vi "tdmstest.vi"   [LabVIEW 2019]
uses:
  TDMSLogger_class/TDMSLogger.lvclass
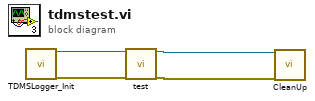
[diagram p0: block diagram]
diagram:
  n1 = call "TDMSLogger_Init.vi"() -> ("object out"=w4:refnum<class "TDMSLogger.lvclass">, "error out"=w3:errorcluster)  [unwired: 17 in, 1 out]
  n2 = call-dynamic "test.vi"("object in"=w4, "error in (no error)"=w3) -> ("object out"=w2:refnum<class "TDMSLogger.lvclass">, "error out"=w1:errorcluster)  [unwired: 16 in]
  n3 = call-dynamic "CleanUp.vi"("object in"=w2, "error in (no error)"=w1) -> ()  [unwired: 16 in, 2 out]
